vi "2 Build No Sail Circle.vi"(9 "Radius":dbl, 11 "UTM Location":T2 {"North" format="%#_10f"; "East" format="%#_8f"}) -> (2 "UTM Circle":T1)   [LabVIEW 2011]
doc: "Turns a UTM location and Radius into a no sail zone, which is a simple cluster with all that info in it."
uses:
  2 Typedefs/UTM Location.ctl
  2 Typedefs/UTM Circle.ctl
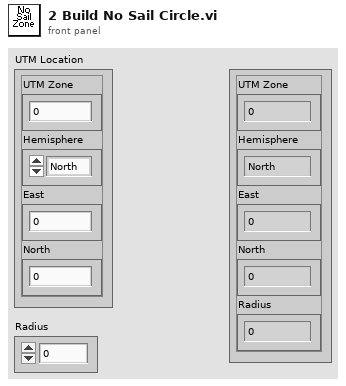
[diagram p1: front panel]
types:
  T1 = typedef "UTM Circle.ctl" = cluster{"UTM Zone":dbl, "Hemisphere":enum16{"North", "South"}, "East":dbl, "North":dbl, "Radius":dbl}
  T2 = typedef "UTM Location.ctl" = cluster{"UTM Zone":dbl, "Hemisphere":enum16{"North", "South"}, "East":dbl, "North":dbl}
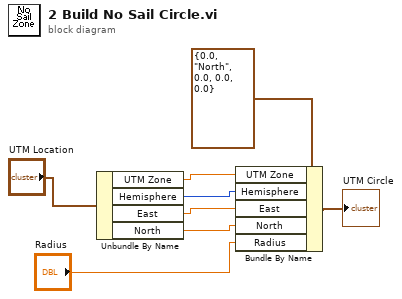
[diagram p0: block diagram]
diagram:
  n1 = Unbundle By Name("UTM Location") -> ("UTM Zone"=w1:dbl, "Hemisphere"=w2:enum16{"North", "South"}, "East"=w3:dbl, "North"=w4:dbl)
  n2 = Bundle By Name(cluster=T1 {"UTM Zone"=0.0, "Hemisphere"=enum."North", "East"=0.0, "North"=0.0, "Radius"=0.0} ("UTM Circle 2"), "UTM Zone"=w1, "Hemisphere"=w2, "East"=w3, "North"=w4, "Radius"="Radius") -> (→"UTM Circle":T1)
